vi "Read Caller-To-Actor Enqueuer.vi"(11 "Last Ack":refnum<class "Last Ack.lvclass">) -> (2 "Caller-to-Actor Enqueuer":refnum<class "Message Enqueuer.lvclass">)   [LabVIEW 2020, in "Actor Framework.lvlib" / "Last Ack.lvclass"]
doc: "<p>(<strong>Filename</strong>: <span class=\"dnl\">Actor Framework.lvlib:Last Ack.lvclass:Read Caller-To-Actor Enqueuer.vi</span>)</p>\n\n<p>Returns the reference the caller used to send messages to the actor. Although the reference is invalid, you can use it to identify which actor shut down.</p>"
uses:
  Last Ack.lvclass
  Message Enqueuer/Message Enqueuer.lvclass
  Last Ack.lvclass/Last Ack.ctl
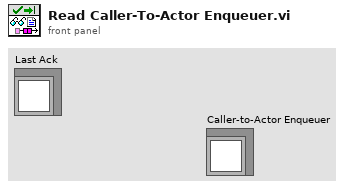
[diagram p1: front panel]
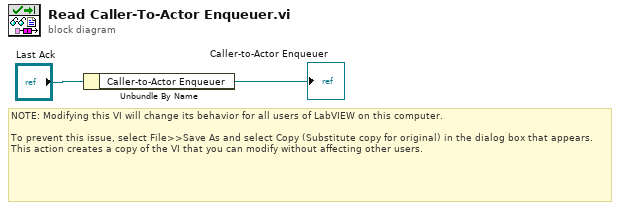
[diagram p0: block diagram]
diagram:
  # "NOTE: Modifying this VI will change its behavior for all users of LabVIEW on this computer.\n\nTo prevent this issue, select File>>Save As and select Copy (Substitute copy for original) in the dialog box that appears. This action creates a copy of the VI that you can modify without affecting other users."
  n1 = Unbundle By Name("Last Ack") -> ("Caller-to-Actor Enqueuer"=→"Caller-to-Actor Enqueuer":refnum<class "Message Enqueuer.lvclass">)
